vi "dfd_Compute Order & Cutoffs.vi"(6 "fs [Hz]":dbl=1.0 format="%.2f", 7 "filter type":T5(ring), 8 "error in (no error)":errorcluster, 9 "design method":T4(ring)=enum."Elliptic", 10 "ripple specs":T2={"passband"=0.1, "stopband"=40.0, "dB/linear? (T: dB)"=TRUE}, 11 "freq specs [Hz]":T3) -> (0 "error out":errorcluster, 1 "low cutoff freq: fl":dbl, 2 "high cutoff freq: fh":dbl, 3 "N":i32=5, 4 "ripples [dB]":T1 {"stopband atten" format="%.2f"; "passband ripple" format="%.2f"})   [LabVIEW 2017, in "NI_DigFilter_Design.lvlib"]
uses:
  <vilib>/addons/Digital Filter Design/NI_DigFilter_Design.lvlib
  <vilib>/addons/Digital Filter Design/_Objects.llb/DFD Filter Frequence Specification (Design).ctl
  <vilib>/addons/Digital Filter Design/_Objects.llb/DFD Filter Ripple Specification (Design).ctl
  <vilib>/Analysis/NI_AAL_Filter.lvlib
  <vilib>/addons/Digital Filter Design/NI_DigFilterLicensed.lvlib
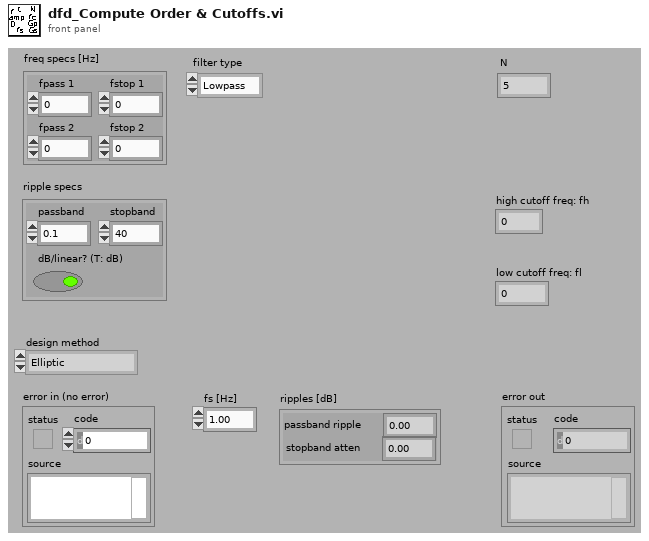
[diagram p1: front panel]
types:
  T1 = cluster{"passband ripple":dbl, "stopband atten":dbl}
  T2 = typedef "NI_DigFilterLicensed.lvlib/DFD Filter Ripple Specification (Design).ctl" = cluster{"passband":dbl, "stopband":dbl, "dB/linear? (T: dB)":bool}
  T3 = typedef "NI_DigFilterLicensed.lvlib/DFD Filter Frequence Specification (Design).ctl" = cluster{"fpass 1":dbl, "fstop 1":dbl, "fpass 2 ":dbl, "fstop 2":dbl}
  T4 = enum16{"Butterworth", "Chebyshev", "Inverse Chebyshev", "Elliptic", "Bessel"}
  T5 = enum16{"Lowpass", "Highpass", "Bandpass", "Bandstop"}
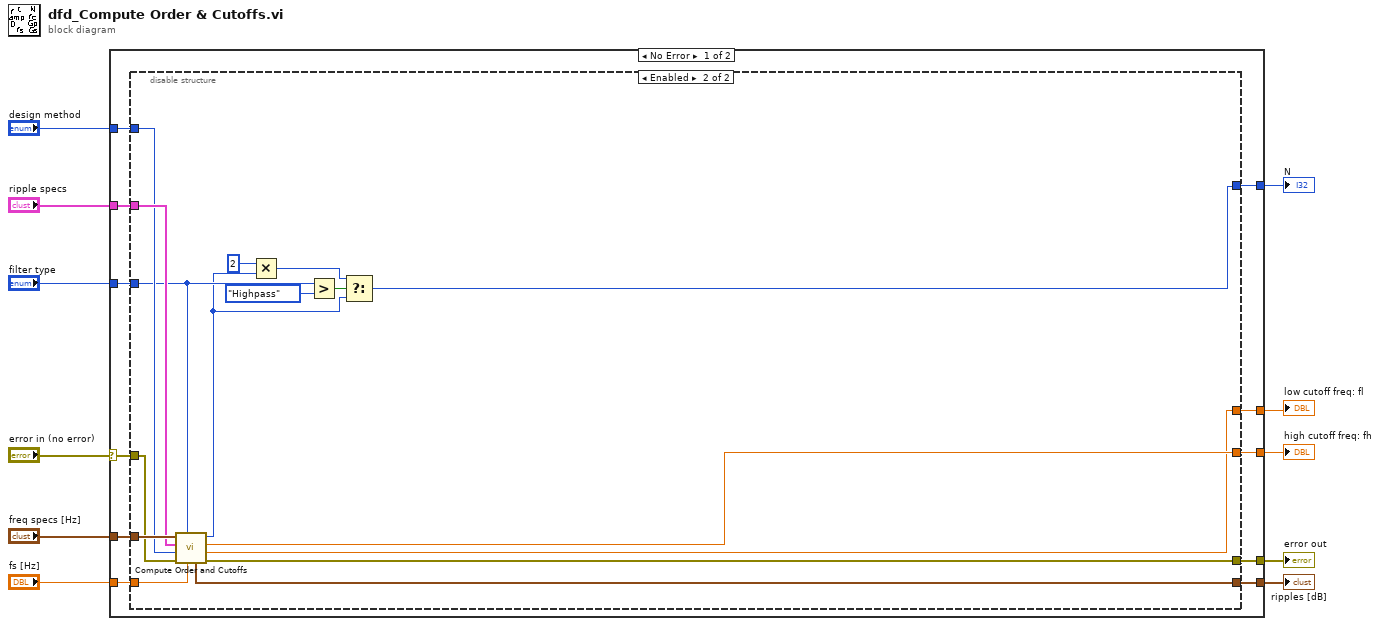
[diagram p0: block diagram]
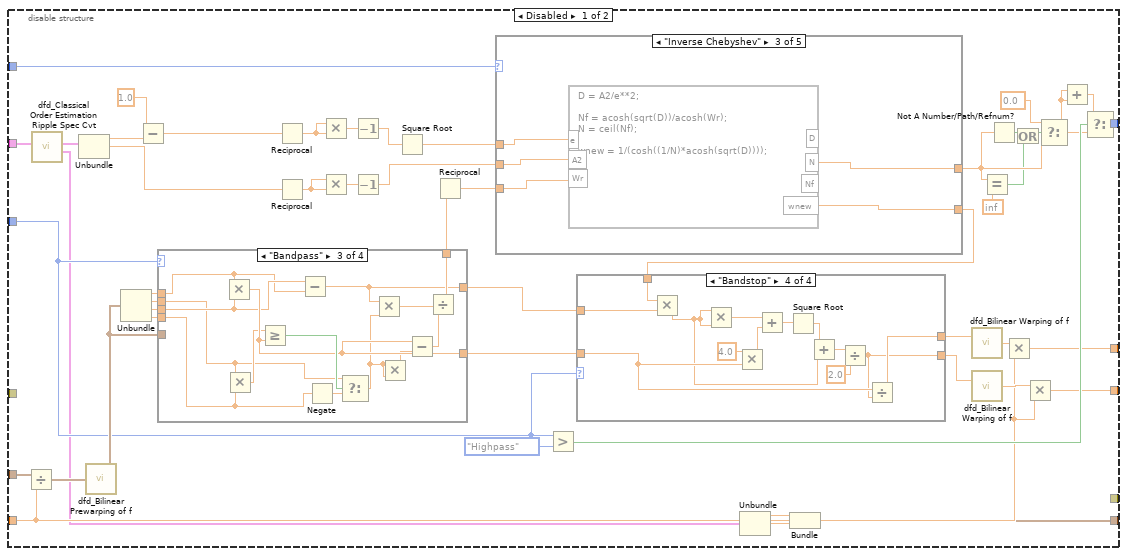
[diagram p2: hidden frame]
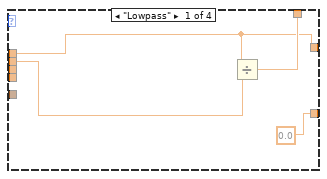
[diagram p3: hidden frame]
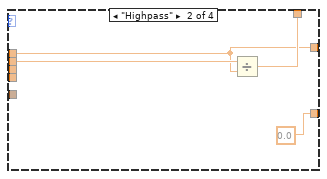
[diagram p4: hidden frame]
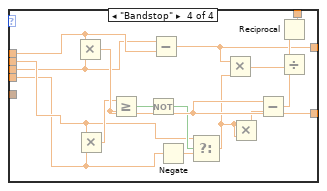
[diagram p5: hidden frame]
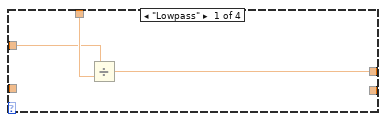
[diagram p6: hidden frame]
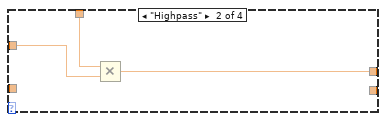
[diagram p7: hidden frame]
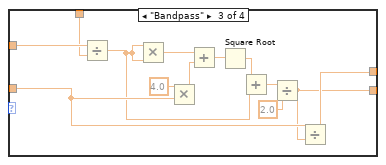
[diagram p8: hidden frame]
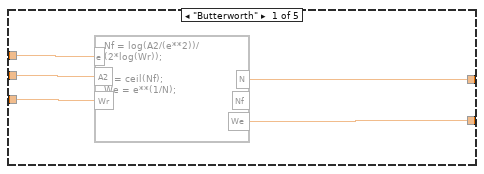
[diagram p9: hidden frame]
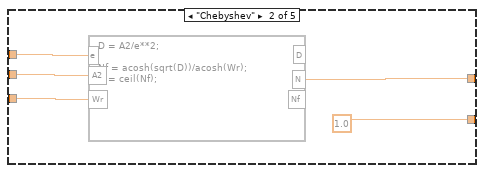
[diagram p10: hidden frame]
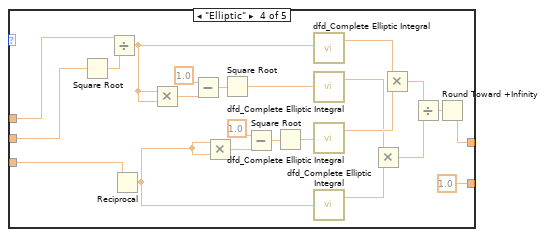
[diagram p11: hidden frame]
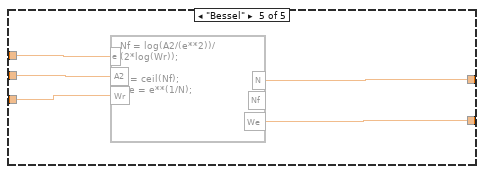
[diagram p12: hidden frame]
diagram:
  n1 = case shown="No Error" "error in (no error)" {
    selector: "error in (no error)" -> [w14 w201]
    tunnel: "filter type" -> [w20 _]
    tunnel: [w19 _] -> w10
    tunnel: "freq specs [Hz]" -> [w22 _]
    tunnel: "fs [Hz]" -> [w17 _]
    tunnel: "ripple specs" -> [w21 _]
    tunnel: [w18 _] -> w5
    tunnel: [w16 _] -> w4
    tunnel: "design method" -> [w15 _]
    tunnel: [w13 _] -> w2
    tunnel: [w12 w201] -> w1
    frame No Error {
      n2 = disable-structure shown="Enabled" {
        disable-tunnel: w22 -> [w53 w200]
        disable-tunnel: w21 -> [w51 w199]
        disable-tunnel: w20 -> [w39 w190]
        disable-tunnel: [w36 w185] -> w19
        disable-tunnel: [w32 w194] -> w18
        disable-tunnel: w17 -> [w29 w197]
        disable-tunnel: [w28 w195] -> w16
        disable-tunnel: w15 -> [w27 w192]
        disable-tunnel: w14 -> [_ w198]
        disable-tunnel: [w23 w196] -> w13
        disable-tunnel: [_ w193] -> w12
        frame Disabled {
          n3 = Divide(x=w53, y=w29) -> (x/y=w47:T3)
          n4 = call <vilib>:"dfd_Classical Order Estimation Ripple Spec Cvt.vi"("ripple specs"=w51) -> ("ripple specs (dB)"=w24:T2, "ripple specs (linear)"=w50:T2)  [unwired: 9 out]
          n5 = Unbundle(w50) -> ("passband"=w49:dbl, "stopband"=w40:dbl)  [unwired: 1 out]
          n6 = call <vilib>:"dfd_Bilinear Prewarping of f.vi"("freq specs [Hz]"=w47) -> ("prewarped freq specs [Hz]"=w46:T3)
          n7 = Unbundle(w46) -> ("fpass 1"=w45:dbl, "fstop 1"=w44:dbl, "fpass 2"=w43:dbl, "fstop 2"=w42:dbl)
          n8 = Subtract(x=1.0, y=w49) -> (x-y=w41:dbl)
          n9 = case shown="\"Bandpass\"" w39 {
            tunnel: [w75 w79 w92 w98] -> w67
            tunnel: [w73 w76 w91 w107] -> w66
            tunnel: [0.0 0.0 w90 w106] -> w65
            tunnel: w46 -> [_ _ _ _]
            tunnel: w45 -> [w73 w76 w80 w97]
            tunnel: w44 -> [w72 w77 w81 w96]
            tunnel: w43 -> [_ _ w83 w95]
            tunnel: w42 -> [_ _ w82 w94]
            frame "Lowpass" {
              n10 = Divide(x=w73, y=w72) -> (x/y=w75:dbl)
            }
            frame "Highpass" {
              n11 = Divide(x=w77, y=w76) -> (x/y=w79:dbl)
            }
            frame "Bandpass" {
              n12 = Multiply(x=w80, y=w83) -> (x*y=w90:dbl)
              n13 = Multiply(x=w81, y=w82) -> (x*y=w89:dbl)
              n14 = Greater Or Equal?(x=w89, y=w90) -> (x >= y?=w93:bool)
              n15 = Subtract(x=w83, y=w80) -> (x-y=w91:dbl)
              n16 = Negate(x=w82) -> (-x=w88:dbl)
              n17 = Select(t=w81, s=w93, f=w88) -> (s? t:f=w87:dbl)
              n18 = Multiply(x=w91, y=w87) -> (x*y=w84:dbl)
              n19 = Multiply(x=w87, y=w87) -> (x*y=w86:dbl)
              n20 = Subtract(x=w90, y=w86) -> (x-y=w85:dbl)
              n21 = Divide(x=w84, y=w85) -> (x/y=w92:dbl)
            }
            frame "Bandstop" {
              n22 = Multiply(x=w97, y=w95) -> (x*y=w106:dbl)
              n23 = Multiply(x=w96, y=w94) -> (x*y=w105:dbl)
              n24 = Greater Or Equal?(x=w105, y=w106) -> (x >= y?=w109:bool)
              n25 = Not(x=w109) -> (.not. x?=w99:bool)
              n26 = Subtract(x=w95, y=w97) -> (x-y=w107:dbl)
              n27 = Negate(x=w94) -> (-x=w104:dbl)
              n28 = Select(t=w96, s=w99, f=w104) -> (s? t:f=w103:dbl)
              n29 = Multiply(x=w107, y=w103) -> (x*y=w100:dbl)
              n30 = Multiply(x=w103, y=w103) -> (x*y=w102:dbl)
              n31 = Subtract(x=w106, y=w102) -> (x-y=w101:dbl)
              n32 = Divide(x=w100, y=w101) -> (x/y=w108:dbl)
              n33 = Reciprocal(x=w108) -> (1/x=w98:dbl)
            }
          }
          n34 = Reciprocal(x=w41) -> (1/x=w60:dbl)
          n35 = Reciprocal(x=w40) -> (1/x=w70:dbl)
          n36 = Multiply(x=w60, y=w60) -> (x*y=w61:dbl)
          n37 = Multiply(x=w70, y=w70) -> (x*y=w69:dbl)
          n38 = Decrement(x=w61) -> (x-1=w62:dbl)
          n39 = Decrement(x=w69) -> (x-1=w71:dbl)
          n40 = Square Root(x=w62) -> (sqrt(x)=w63:dbl)
          n41 = Reciprocal(x=w67) -> (1/x=w68:dbl)
          n42 = case shown="\"Inverse Chebyshev\"" w27 {
            tunnel: w68 -> [w146 w150 w155 w158 w184]
            tunnel: [w145 1.0 w152 1.0 w183] -> w64
            tunnel: w63 -> [w144 w149 w154 w161 w182]
            tunnel: [w142 w147 w153 w160 w181] -> w57
            tunnel: w71 -> [w143 w151 w156 w157 w180]
            frame "Butterworth" {
              n43 = formula code="Nf = log(A2/(e**2))/\n(2*log(Wr));\n\nN = ceil(Nf);\nWe = e**(1/N);"("e"=w144, "A2"=w143, "Wr"=w146) -> ("N"=w142:dbl, "We"=w145:dbl)  [unwired: 1 out]
            }
            frame "Chebyshev" {
              n44 = formula code="D = A2/e**2;\n\nNf = acosh(sqrt(D))/acosh(Wr);\nN = ceil(Nf);"("e"=w149, "A2"=w151, "Wr"=w150) -> ("N"=w147:dbl)  [unwired: 2 out]
            }
            frame "Inverse Chebyshev" {
              n45 = formula code="D = A2/e**2;\n\nNf = acosh(sqrt(D))/acosh(Wr);\nN = ceil(Nf);\n\nwnew = 1/(cosh((1/N)*acosh(sqrt(D))));"("e"=w154, "A2"=w156, "Wr"=w155) -> ("N"=w153:dbl, "wnew"=w152:dbl)  [unwired: 2 out]
            }
            frame "Elliptic" {
              n46 = Square Root(x=w157) -> (sqrt(x)=w179:dbl)
              n47 = Divide(x=w161, y=w179) -> (x/y=w171:dbl)
              n48 = Reciprocal(x=w158) -> (1/x=w162:dbl)
              n49 = Multiply(x=w171, y=w171) -> (x*y=w173:dbl)
              n50 = Subtract(x=1.0, y=w173) -> (x-y=w174:dbl)
              n51 = Multiply(x=w162, y=w162) -> (x*y=w177:dbl)
              n52 = Square Root(x=w174) -> (sqrt(x)=w170:dbl)
              n53 = Subtract(x=1.0, y=w177) -> (x-y=w176:dbl)
              n54 = Square Root(x=w176) -> (sqrt(x)=w175:dbl)
              n55 = call <vilib>:"dfd_Complete Elliptic Integral.vi"("k'"=w171) -> ("cei(k)"=w169:dbl)  [unwired: 1 out]
              n56 = call <vilib>:"dfd_Complete Elliptic Integral.vi"("k'"=w170) -> ("cei(k)"=w163:dbl)  [unwired: 1 out]
              n57 = call <vilib>:"dfd_Complete Elliptic Integral.vi"("k'"=w175) -> ("cei(k)"=w168:dbl)  [unwired: 1 out]
              n58 = call <vilib>:"dfd_Complete Elliptic Integral.vi"("k'"=w162) -> ("cei(k)"=w167:dbl)  [unwired: 1 out]
              n59 = Multiply(x=w163, y=w167) -> (x*y=w166:dbl)
              n60 = Multiply(x=w169, y=w168) -> (x*y=w165:dbl)
              n61 = Divide(x=w165, y=w166) -> (x/y=w164:dbl)
              n62 = Round Toward +Infinity(x=w164) -> (ceil(x): smallest int >= x=w160:dbl)
            }
            frame "Bessel" {
              n63 = formula code="Nf = log(A2/(e**2))/\n(2*log(Wr));\n\nN = ceil(Nf);\nWe = e**(1/N);"("e"=w182, "A2"=w180, "Wr"=w184) -> ("N"=w181:dbl, "We"=w183:dbl)  [unwired: 1 out]
            }
          }
          n64 = Greater?(x=w39, y=T5."Highpass") -> (0:w37:bool)
          n65 = case shown="\"Bandstop\"" w39 {
            tunnel: w66 -> [w111 w114 w128 w132]
            tunnel: w65 -> [_ _ w127 w141]
            tunnel: w64 -> [w112 w115 w120 w131]
            tunnel: [w110 w113 w117 w130] -> w33
            tunnel: [_ _ w116 w129] -> w30
            frame "Lowpass" {
              n66 = Divide(x=w111, y=w112) -> (x/y=w110:dbl)
            }
            frame "Highpass" {
              n67 = Multiply(x=w115, y=w114) -> (x*y=w113:dbl)
            }
            frame "Bandpass" {
              n68 = Divide(x=w128, y=w120) -> (x/y=w118:dbl)
              n69 = Multiply(x=w118, y=w118) -> (x*y=w119:dbl)
              n70 = Multiply(x=4.0, y=w127) -> (x*y=w122:dbl)
              n71 = Add(x=w119, y=w122) -> (x+y=w123:dbl)
              n72 = Square Root(x=w123) -> (sqrt(x)=w124:dbl)
              n73 = Add(x=w124, y=w118) -> (x+y=w125:dbl)
              n74 = Divide(x=w125, y=2.0) -> (x/y=w116:dbl)
              n75 = Divide(x=w127, y=w116) -> (x/y=w117:dbl)
            }
            frame "Bandstop" {
              n76 = Multiply(x=w131, y=w132) -> (x*y=w133:dbl)
              n77 = Multiply(x=w133, y=w133) -> (x*y=w134:dbl)
              n78 = Multiply(x=4.0, y=w141) -> (x*y=w136:dbl)
              n79 = Add(x=w134, y=w136) -> (x+y=w137:dbl)
              n80 = Square Root(x=w137) -> (sqrt(x)=w138:dbl)
              n81 = Add(x=w138, y=w133) -> (x+y=w139:dbl)
              n82 = Divide(x=w139, y=2.0) -> (x/y=w129:dbl)
              n83 = Divide(x=w141, y=w129) -> (x/y=w130:dbl)
            }
          }
          n84 = Unbundle(w24) -> ("passband"=w25:dbl, "stopband"=w26:dbl)  [unwired: 1 out]
          n85 = Bundle("passband"=w25, "stopband"=w26) -> (w23:cluster{"passband":dbl, "stopband":dbl})  [unwired: 1 out]
          n86 = call <vilib>:"dfd_Bilinear Warping of f.vi"("f"=w33) -> ("prewarped f"=w52:dbl)
          n87 = call <vilib>:"dfd_Bilinear Warping of f.vi"("f"=w30) -> ("prewarped f"=w31:dbl)
          n88 = Equal?(x=w57, y=inf) -> (x = y?=w54:bool)
          n89 = Not A Number/Path/Refnum?(number/path/refnum=w57) -> (NaN/Path/Refnum?=w59:bool)
          n90 = Multiply(x=w52, y=w29) -> (x*y=w32:dbl)
          n91 = Or(x=w59, y=w54) -> (x .or. y?=w55:bool)
          n92 = Multiply(x=w31, y=w29) -> (x*y=w28:dbl)
          n93 = Select(t=0.0, s=w55, f=w57) -> (s? t:f=w34:dbl)
          n94 = Add(x=w34, y=w34) -> (x+y=w35:dbl)
          n95 = Select(t=w35, s=w37, f=w34) -> (s? t:f=w36:dbl)
        }
        frame Enabled {
          n96 = call <vilib>:"Compute Order and Cutoffs.vi"("fs [Hz]"=w197, "filter type"=w190, "error in (no error)"=w198, "design method"=w192, "ripple specs"=w199, "freq specs [Hz]"=w200) -> ("error out"=w193:errorcluster, "low cutoff freq: fl"=w194:dbl, "high cutoff freq: fh"=w195:dbl, "n"=w188:i32, "ripples [dB]"=w196:T1)  [unwired: 1 in]
          n97 = Multiply(x=2, y=w188) -> (x*y=w186:i32)
          n98 = Greater?(x=w190, y=T5."Highpass" ("filter type")) -> (0:w189:bool)
          n99 = Select(t=w186, s=w189, f=w188) -> (s? t:f=w185:i32)
        }
      }
    }
    frame Error {
    }
  }
  "N" <- w10
  "error out" <- w1
  "ripples [dB]" <- w2
  "low cutoff freq: fl" <- w5
  "high cutoff freq: fh" <- w4
